vi "Write w12 LP IIR coeffs.vi"(9 "Fs [MHz}":dbl min=0.0 max=1.0, 10 "cutoff fequency [MHz]":dbl min=0.0 max=10000.0, 11 "FpgaRef5761":refnum<class "FpgaRef5761.lvclass">) -> (3 "FpgaRef5761":refnum<class "FpgaRef5761.lvclass">)   [LabVIEW 2018]
uses:
  FpgaRef/FpgaRef5761/FpgaRef5761.lvclass
  E:/PXIe/in progress/source/Host/FpgaRef/FpgaRefBase/FpgaRefBase.lvclass
  FPGA/fpga_settings.ctl
  <vilib>/rvi/FXPMathLib/FxpInterpret/XNode/nifxpmath_Interpret.xnode
  FpgaRef/FpgaRefBase/FpgaRefBase.lvclass
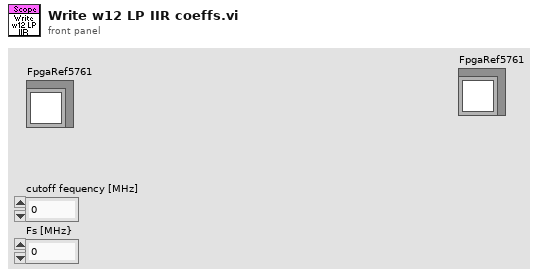
[diagram p1: front panel]
types:
  T1 = typedef "fpga_settings.ctl" = enum16{"Feedback Enable", "New FIR coeffs", "FIR shift", "Enable filter", "Set Downsample", "Downsample", "CIC Gain", "Record length", "Trigger samples", "Quiet time", "a_am", "b_am", "Use fixed delay", "fixed sin_fi", "fixed cos_fi", "Ki*Tau", "Kp", "Kd_Tau", "Fi_start", "Fi_delta", "DC_offs 0", "DC_offs 1", "DC_offs 2", "DC_offs 3", "Ki*Tau am", "Kp am", "Kd_Tau am", "Feedback AM", "Trigger delay", "Feedback delay", "Setpoint enable", "Beam enable", "Samples to acquire", "Cavity Enable", "Cavity C1", "Cavity C2", "Cavity C3", "Cavity C4", "Cavity C5", "Input delay", "Ki*Tau Q", "Kp Q", "Kd_Tau Q", "Adaptive FF enable", "Feedforward a0", "Feedforward b0", "FF src adress", "FF dest adress", "Output scale", "Input scale", "Host scale", "FF_IIR b0", "FF_IIR b1", "FF_IIR b2", "FF_IIR-a1", "FF_IIR-a2", "Enable HW trigger", "Virtual cavity", "Samples to skip", "Samples to skip 2", "Samples to skip 3", "Cavity C3_2", "Cavity C4_2", "Cavity C5_2", "Cavity C3_3", "Cavity C4_3", "Cavity C5_3", "Cavity_w0_dt", "Piezo setting", "Quench t0", "Quench tau set", "Quench enabled", "Quench reset", "PID enabled I", "PID enabled Q", "Cavity filter a", "Cavity filter b", "Disable e(n)", "FF e(n) src address", "FF first address", "FF last address", "FF PID first address", "FF PID last address", "Amp IIR b0", "Amp IIR b1", "Amp IIR b2", "Amp IIR-a1", "Amp IIR-a2", "Adaptation factor", "Inv Amp LP b0", "Inv Amp LP b1", "Inv Amp LP b2", "Inv Amp LP-a1", "Inv Amp LP-a2", "Inv Amp c0", "Inv Amp c1", "Inv Amp c2", "Inv Amp c3", "Inv Amp c4", "Inv Amp -d1", "Inv Amp -d2", "Inv Amp -d3", "Inv Amp -d4", "w12_a", "w12_b", "w12_dt", "w12_scale", "dw_scale"}
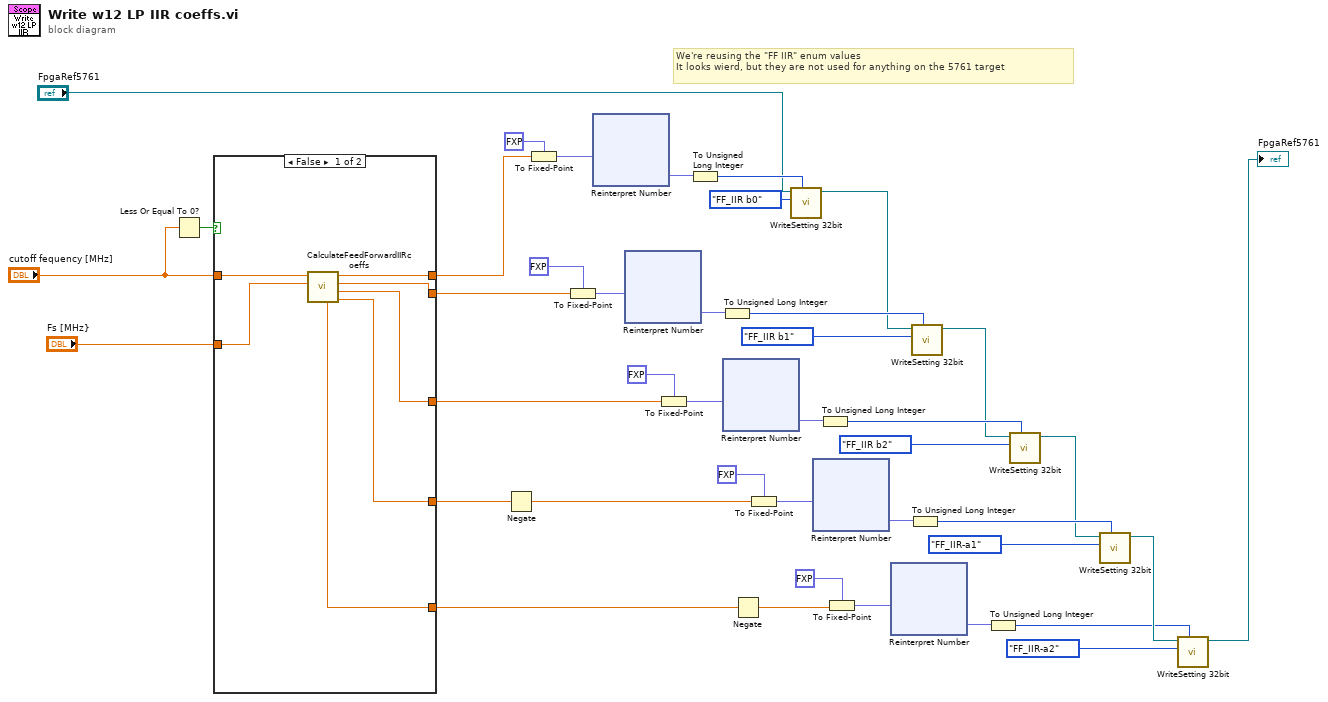
[diagram p0: block diagram]
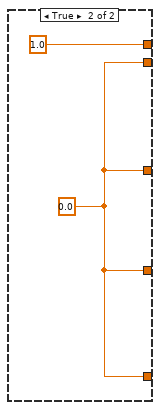
[diagram p2: hidden frame]
diagram:
  # "We're reusing the \"FF IIR\" enum values\nIt looks wierd, but they are not used for anything on the 5761 target"
  n1 = Less Or Equal To 0?(x="cutoff fequency [MHz]") -> (x <= 0?=w1:bool)
  n2 = case shown="False" w1 {
    tunnel: "cutoff fequency [MHz]" -> [w48 _]
    tunnel: "Fs [MHz}" -> [w47 _]
    tunnel: [w46 1.0 ("b0")] -> w30
    tunnel: [w45 w49] -> w28
    tunnel: [w44 w49] -> w9
    tunnel: [w43 w49] -> w8
    tunnel: [w42 w49] -> w6
    frame False {
      n3 = call "CalculateFeedForwardIIRcoeffs.vi"("fs [MHz]"=w47, "fc [MHz]"=w48) -> ("a1"=w43:dbl, "b2"=w44:dbl, "b1"=w45:dbl, "b0"=w46:dbl, "a2"=w42:dbl)  [unwired: 5 in]
    }
    frame True {
      w49 = 0.0 ("b0")
    }
  }
  n4 = Negate(x=w8) -> (-x=w7:dbl)
  n5 = To Fixed-Point(fixed-point type=fxp<+/-,32,2> 0.0 ("x"), number=w30) -> (fixed-point=w40:fxp<+/-,32,2>)
  n6 = To Fixed-Point(fixed-point type=fxp<+/-,32,2> 0.0 ("x"), number=w28) -> (fixed-point=w34:fxp<+/-,32,2>)
  n7 = xnode "Reinterpret Number"("x"=w40) -> ("y"=w41:fxp<+,32,32>)
  n8 = xnode "Reinterpret Number"("x"=w34) -> ("y"=w33:fxp<+,32,32>)
  n9 = To Fixed-Point(fixed-point type=fxp<+/-,32,2> 0.0 ("x"), number=w9) -> (fixed-point=w25:fxp<+/-,32,2>)
  n10 = To Unsigned Long Integer(number=w41) -> (unsigned 32bit integer=w39:u32)
  n11 = To Unsigned Long Integer(number=w33) -> (unsigned 32bit integer=w36:u32)
  n12 = xnode "Reinterpret Number"("x"=w25) -> ("y"=w26:fxp<+,32,32>)
  n13 = Negate(x=w6) -> (-x=w3:dbl)
  n14 = To Fixed-Point(fixed-point type=fxp<+/-,32,2> 0.0 ("x"), number=w7) -> (fixed-point=w18:fxp<+/-,32,2>)
  n15 = call "WriteSetting 32bit.vi"("value"=w39, "FPGA Setting"=fpga_settings."FF_IIR b0", "FpgaRefBase in"="FpgaRef5761") -> ("FpgaRefBase out"=w32:refnum<class "FpgaRef5761.lvclass">)  [unwired: 7 in, 1 out]
  n16 = xnode "Reinterpret Number"("x"=w18) -> ("y"=w17:fxp<+,32,32>)
  n17 = To Unsigned Long Integer(number=w26) -> (unsigned 32bit integer=w23:u32)
  n18 = To Fixed-Point(fixed-point type=fxp<+/-,32,2> 0.0 ("x"), number=w3) -> (fixed-point=w4:fxp<+/-,32,2>)
  n19 = xnode "Reinterpret Number"("x"=w4) -> ("y"=w16:fxp<+,32,32>)
  n20 = To Unsigned Long Integer(number=w17) -> (unsigned 32bit integer=w20:u32)
  n21 = call "WriteSetting 32bit.vi"("value"=w36, "FPGA Setting"=fpga_settings."FF_IIR b1", "FpgaRefBase in"=w32) -> ("FpgaRefBase out"=w13:refnum<class "FpgaRef5761.lvclass">)  [unwired: 7 in, 1 out]
  n22 = To Unsigned Long Integer(number=w16) -> (unsigned 32bit integer=w5:u32)
  n23 = call "WriteSetting 32bit.vi"("value"=w23, "FPGA Setting"=fpga_settings."FF_IIR b2", "FpgaRefBase in"=w13) -> ("FpgaRefBase out"=w12:refnum<class "FpgaRef5761.lvclass">)  [unwired: 7 in, 1 out]
  n24 = call "WriteSetting 32bit.vi"("value"=w20, "FPGA Setting"=fpga_settings."FF_IIR-a1", "FpgaRefBase in"=w12) -> ("FpgaRefBase out"=w11:refnum<class "FpgaRef5761.lvclass">)  [unwired: 7 in, 1 out]
  n25 = call "WriteSetting 32bit.vi"("value"=w5, "FPGA Setting"=fpga_settings."FF_IIR-a2", "FpgaRefBase in"=w11) -> ("FpgaRefBase out"=→"FpgaRef5761":refnum<class "FpgaRef5761.lvclass">)  [unwired: 7 in, 1 out]
